vi "RT Network Stream.vi"(11 "Queue ref":T1) -> ()   [LabVIEW 2022 SP3]
uses:
  RT Controls/RT All Queue.ctl
  RT Controls/RT Network Stream.ctl
  RT Controls/RT All Loop Status.ctl
  RT Sub VI's/RT Global.vi
panel:
  out "error out":errorcluster
  out "x != 0?":bool
  out "Status List Out":bool[](array[boolean])
  in  "error in":errorcluster
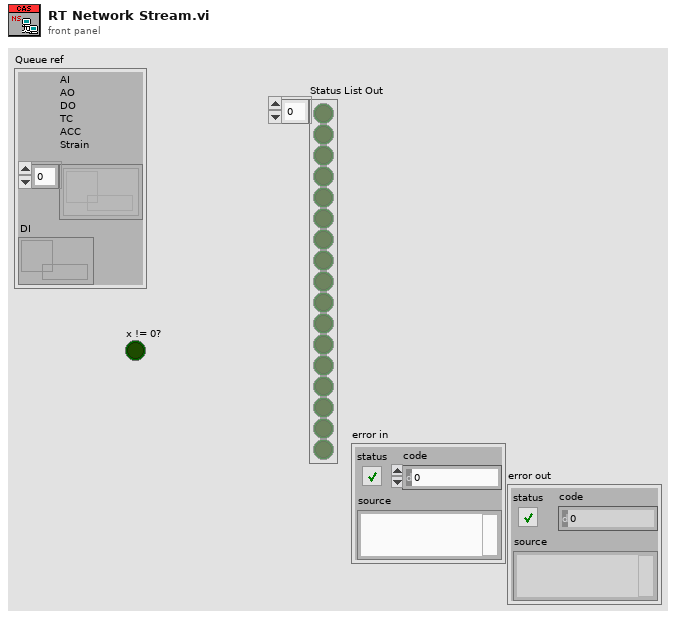
[diagram p1: front panel]
types:
  T1 = typedef "RT All Queue.ctl" = cluster{"AI\nAO\nDO\nTC\nACC\nStrain":refnum<queue>[], "DI":refnum<queue>}
  T2 = cluster{"in progress?":bool, "Exit":bool, "Writer URL":refnum<k21>, "reader url":refnum<k21>, "Queue ref":T1}
  T3 = typedef "RT Network Stream.ctl" = enum16{"Initialize", "Wait For Connection", "Receive Command", "Send Data ", "Flush Data", "Exit"}
  T4 = enum16{"Init", "Read 'All'", "Read 'n'", "Read '1'", "Write '1'", "Write 'n'", "Write 'All'"}
  T5 = typedef "RT All Loop Status.ctl" = enum16{"AI", "AO", "DI", "DO", "TC", "Strain", "ACC", "RT", "Log", "Seq"}
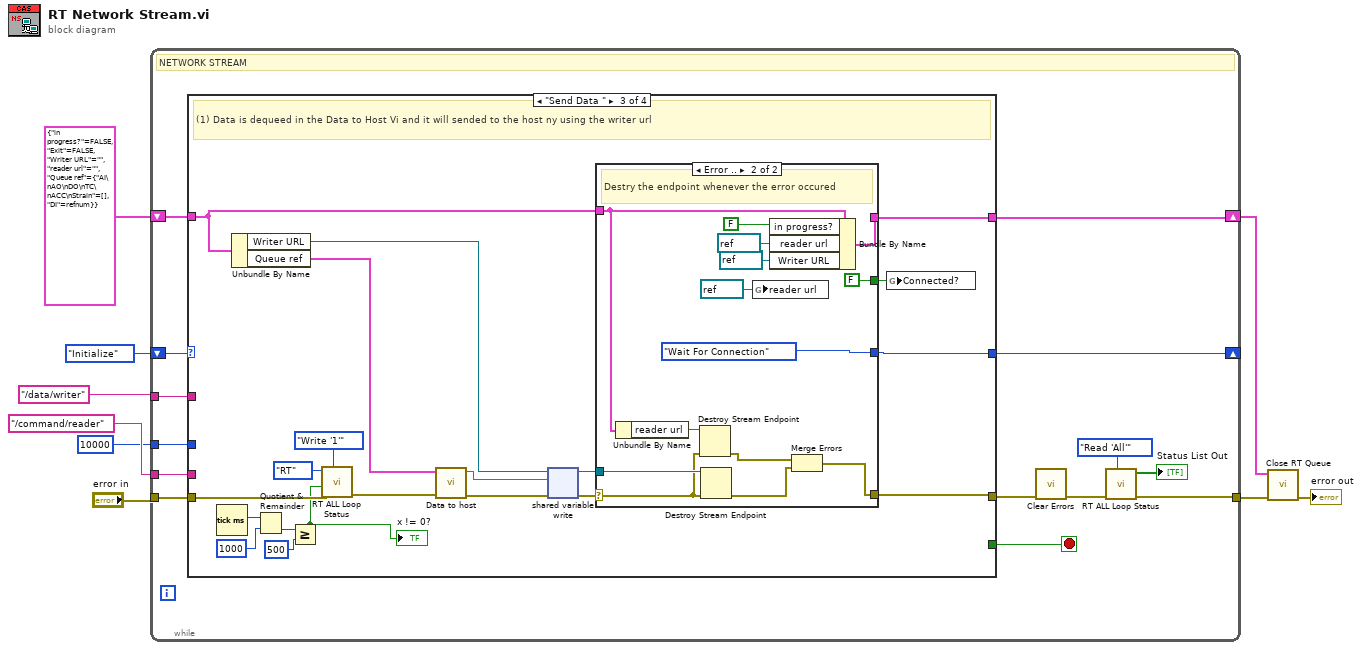
[diagram p0: block diagram]
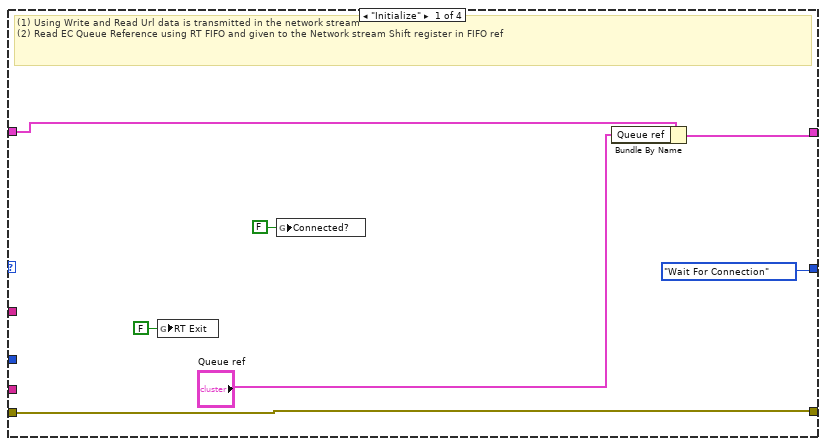
[diagram p2: hidden frame]
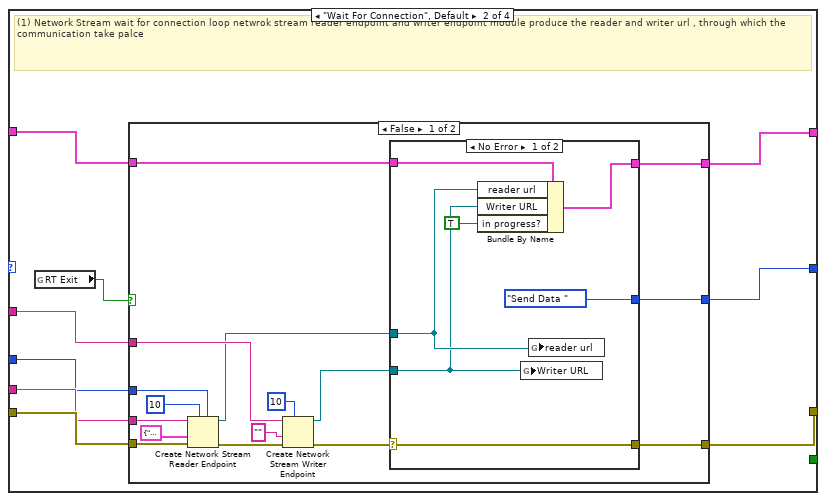
[diagram p3: hidden frame]
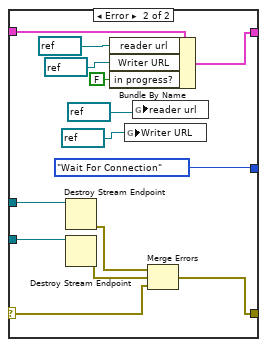
[diagram p4: hidden frame]
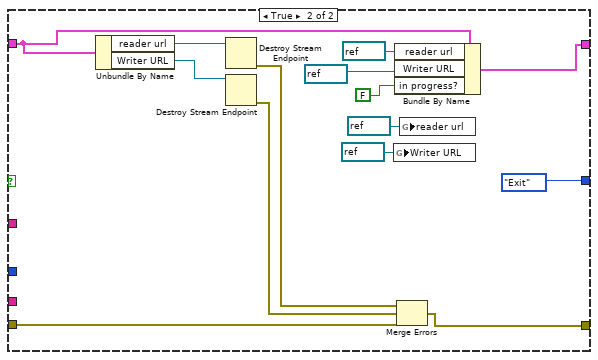
[diagram p5: hidden frame]
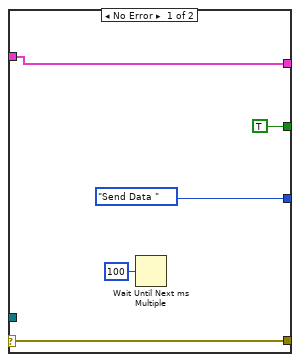
[diagram p6: hidden frame]
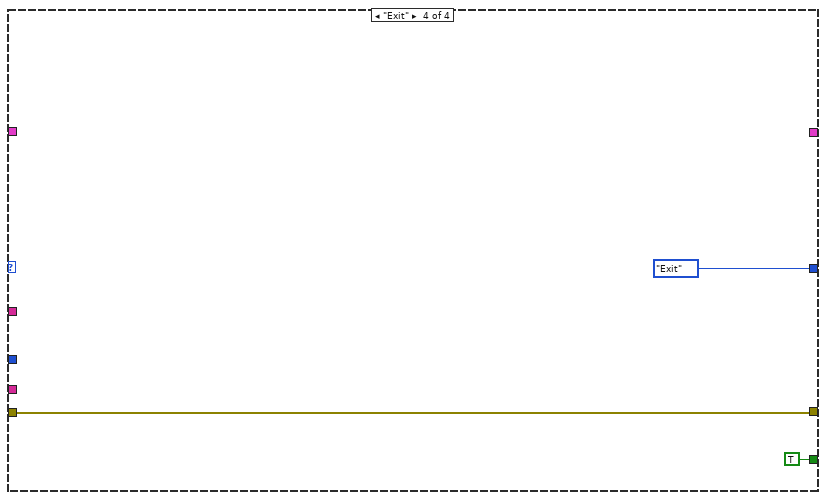
[diagram p7: hidden frame]
diagram:
  n1 = while {
    shift-right: [w22] -> _
    shift-left: RT_Network_Stream."Initialize" -> [w23]
    tunnel: "/command/reader" ("reader url") -> [w20]
    tunnel: "/data/writer" ("reader url") -> [w19]
    tunnel: 10000 ("timeout in ms (-1)") -> [w18]
    shift-right: [w16] -> w2
    shift-left: T2 {"in progress?"=FALSE, "Exit"=FALSE, "Writer URL"="", "reader url"="", "Queue ref"={"AI\nAO\nDO\nTC\nACC\nStrain"=[], "DI"=refnum}} -> [w15]
    tunnel: "error in" -> [w21]
    tunnel: [w13] -> w3
    stop <- w17 stop-if-true
    # "NETWORK STREAM"
    n2 = case shown="\"Send Data \"" w23 {
      tunnel: [RT_Network_Stream."Wait For Connection" w35 w109 RT_Network_Stream."Exit"] -> w22
      tunnel: [w25 w32 w110 w131] -> w14
      tunnel: w21 -> [w25 w39 w101 w131]
      tunnel: w20 -> [_ w38 _ _]
      tunnel: w19 -> [_ w37 _ _]
      tunnel: w18 -> [_ w36 _ _]
      tunnel: w15 -> [w29 w33 w107 _]
      tunnel: [w30 w34 w108 _] -> w16
      tunnel: [_ _ _ TRUE] -> w17
      frame "Initialize" {
        # "(1) Using Write and Read Url data is transmitted in the network stream\n(2) Read EC Queue Reference using RT FIFO and given to the Network stream Shift register in FIFO ref"
        n3 = global write "RT Global.vi" "RT Exit"(FALSE ("RT Exit")) -> ()
        n4 = global write "RT Global.vi" "Connected?"(FALSE ("Connected?")) -> ()
        n5 = Bundle By Name(cluster=w29, "Queue ref"="Queue ref") -> (w30:T2)
      }
      frame "Wait For Connection", Default {
        # "(1) Network Stream wait for connection loop netwrok stream reader endpoint and writer endpoint module produce the reader and writer url , through which the communication take palce"
        n6 = global read "RT Global.vi" "RT Exit"() -> (w31:bool)
        n7 = case shown="False" w31 {
          tunnel: w39 -> [w55 w81]
          tunnel: w38 -> [w53 _]
          tunnel: w37 -> [w52 _]
          tunnel: w36 -> [w40 _]
          tunnel: [w41 w78] -> w32
          tunnel: [w46 RT_Network_Stream."Exit"] -> w35
          tunnel: [w45 w88] -> w34
          tunnel: w33 -> [w44 w87]
          frame False {
            n8 = Create Network Stream Reader Endpoint(5:w40, 7:10 ("reader buffer size"), 8:w55, 9:cluster{"Message":string, "Data":variant} {"Message"="", "Data"=variant}, 11:w53) -> (0:w54:errorcluster, 3:w50:refnum<k21>)  [unwired: 2 in]
            n9 = Create Network Stream Writer Endpoint(7:10 ("reader buffer size"), 8:w54, 9:"" ("data out"), 11:w52) -> (0:w51:errorcluster, 3:w49:refnum<k21>)  [unwired: 3 in]
            n10 = case shown="No Error" w51 {
              selector: w51 -> [w59 w67]
              tunnel: w50 -> [w57 w74]
              tunnel: w49 -> [w56 w73]
              tunnel: [RT_Network_Stream."Send Data " RT_Network_Stream."Wait For Connection"] -> w46
              tunnel: w44 -> [w62 w76]
              tunnel: [w61 w75] -> w45
              tunnel: [w59 w66] -> w41
              frame No Error {
                n11 = Bundle By Name(cluster=w62, "reader url"=w57, "Writer URL"=w56, "in progress?"=TRUE) -> (w61:T2)
                n12 = global write "RT Global.vi" "Writer URL"(w56) -> ()
                n13 = global write "RT Global.vi" "reader url"(w57) -> ()
              }
              frame Error {
                n14 = Destroy Stream Endpoint(11:w74) -> (0:w69:errorcluster)  [unwired: 1 in]
                n15 = Destroy Stream Endpoint(11:w73) -> (0:w68:errorcluster)  [unwired: 1 in]
                n16 = Bundle By Name(cluster=w76, "reader url"=refnum<k21> refnum, "Writer URL"=refnum<k21> refnum, "in progress?"=FALSE) -> (w75:T2)
                n17 = global write "RT Global.vi" "Writer URL"(refnum<k21> refnum ("Writer URL")) -> ()
                n18 = global write "RT Global.vi" "reader url"(refnum<k21> refnum ("reader url")) -> ()
                n19 = Merge Errors(w69, w68, w67) -> (w66:errorcluster)
              }
            }
          }
          frame True {
            n20 = Unbundle By Name(w87) -> ("reader url"=w90:refnum<k21>, "Writer URL"=w89:refnum<k21>)
            n21 = Destroy Stream Endpoint(11:w90) -> (0:w79:errorcluster)  [unwired: 1 in]
            n22 = Destroy Stream Endpoint(11:w89) -> (0:w80:errorcluster)  [unwired: 1 in]
            n23 = global write "RT Global.vi" "Writer URL"(refnum<k21> refnum ("Writer URL")) -> ()
            n24 = Bundle By Name(cluster=w87, "reader url"=refnum<k21> refnum, "Writer URL"=refnum<k21> refnum, "in progress?"=FALSE) -> (w88:T2)
            n25 = Merge Errors(w79, w80, w81) -> (w78:errorcluster)
            n26 = global write "RT Global.vi" "reader url"(refnum<k21> refnum ("reader url")) -> ()
          }
        }
      }
      frame "Send Data " {
        # "(1) Data is dequeed in the Data to Host Vi and it will sended to the host ny using the writer url"
        n27 = Tick Count (ms)() -> (millisecond timer value=w95:u32)
        n28 = Unbundle By Name(w107) -> ("Writer URL"=w105:refnum<k21>, "Queue ref"=w96:T1)
        n29 = Quotient & Remainder(x=w95, y=u32 1000) -> (x-y*floor(x/y)=w93:u32)  [unwired: 1 out]
        n30 = Greater Or Equal?(x=w93, y=u32 500) -> (x >= y?=w91:bool)
        "x != 0?" <- w91
        n31 = call "RT ALL Loop Status.vi"("Option"=T4."Write '1'", "error in (no error)"=w101, "Status"=w91, "Loop"=RT_All_Loop_Status."RT") -> ("error out"=w100:errorcluster)  [unwired: 5 in, 2 out]
        n32 = call "Data to host.vi"("error in"=w100, "Queue ref"=w96) -> ("error out"=w103:errorcluster, "data to Host"=w102:string)  [unwired: 8 in]
        n33 = shared-variable-write(w105, w103, w102) -> (w104:refnum<k21>, w106:errorcluster)  [unwired: 1 in, 1 out]
        n34 = case shown="Error .." w106 {
          selector: w106 -> [w115 w118]
          tunnel: [w115 w117] -> w110
          tunnel: [RT_Network_Stream."Send Data " RT_Network_Stream."Wait For Connection"] -> w109
          tunnel: [w114 w129] -> w108
          tunnel: w107 -> [w114 w126]
          tunnel: w104 -> [_ w127]
          tunnel: [TRUE FALSE] -> w97
          frame No Error {
            n35 = Wait Until Next ms Multiple(millisecond multiple=u32 100) -> ()  [unwired: 1 out]
          }
          frame Error {
            # "Destry the endpoint whenever the error occured"
            n36 = Unbundle By Name(w126) -> ("reader url"=w125:refnum<k21>)
            n37 = Destroy Stream Endpoint(8:w118, 11:w125) -> (0:w120:errorcluster)
            n38 = Destroy Stream Endpoint(8:w118, 11:w127) -> (0:w119:errorcluster)
            n39 = global write "RT Global.vi" "reader url"(refnum<k21> refnum ("reader url")) -> ()
            n40 = Bundle By Name(cluster=w126, "in progress?"=FALSE, "reader url"=refnum<k21> refnum, "Writer URL"=refnum<k21> refnum) -> (w129:T2)
            n41 = Merge Errors(w120, w119) -> (w117:errorcluster)
          }
        }
        n42 = global write "RT Global.vi" "Connected?"(w97) -> ()
      }
      frame "Exit" {
      }
    }
    n43 = call <vilib>:"Clear Errors.vi"("error in (no error)"=w14) -> ("error out"=w10:errorcluster)  [unwired: 5 in, 1 out]
    n44 = call "RT ALL Loop Status.vi"("Option"=T4."Read 'All'", "error in (no error)"=w10) -> ("error out"=w13:errorcluster, "Status List Out"=→"Status List Out":bool[])  [unwired: 7 in, 1 out]
  }
  n45 = call "Close RT Queue.vi"("error in"=w3, "queue"=w2) -> ("error out"=→"error out":errorcluster)  [unwired: 9 in]
